vi "Y Translation Test.vi"() -> ()   [LabVIEW 2020]
doc: "This example performs writes and reads on a serial port, as directed by the user. You can press the Write and Read buttons, and change the Read Count, while the example is running.\n\nThe parameters set for the serial port must match the parameters of the connected instrument or device. In this example, the Read Count parameter specifies the number of bytes that the serial port reads. If there were more bytes at the port than the specified number, those bytes would not be read. If there were less bytes at the port than the specified number, you would receive a timeout error.\n\nThis example expands upon the flow control options for XON and XOFF, allowing the user to choose those control characters. Also, the user can enable or disable a termination character. Some devices require a termination character in order to identify the end of command strings. Some devices send a termination character to signify the end of data to be read. This example shows how you can end the Read operation once a termination character is detected in the buffer and/or append a termination character at the end of the Write data."
uses:
  Program Files/National Instruments/LabVIEW 2020/examples/Instrument IO/Serial/support/Serial - Settings.ctl
  <vilib>/Instr/_visa.llb/VISA Configure Serial Port (Instr).vi
panel:
  out "read buffer":string
  out "Limit Switch Activated":bool
  out "Moving":bool
  out "Boolean array":bool[](array[boolean])
  out "Number":i32
  out "Binary Number":i32=2374 format="%b"
  in  "Stop":bool
  in  "Command":string="@01 AMOV 200"
  in  "Send":bool
  in  "Serial Settings":T1={"baud rate"=57600, "data bits"=8, "parity"=enum."None", "stop bits"=10, "flow control"=0} {"flow control" items=["None"=0, "XON/XOFF"=1, "RTS/CTS"=2, "DTR/DSR"=4]; "stop bits" items=["1.0"=10, "1.5"=15, "2.0"=20]; "data bits" min=5 max=8 step=1; "baud rate" items=["75"=75, "110"=110, "134"=134, "150"=150, "300"=300, "600"=600, "1200"=1200, "1800"=1800, "2400"=2400, "4800"=4800, "7200"=7200, "9600"=9600, "14400"=14400, "19200"=19200, "28800"=28800, "38400"=38400, "56000"=56000, "57600"=57600, "115200"=115200, "128000"=128000, "230400"=230400]}
  in  "VISA resource name":refnum<visa-resource-name>="COM3"
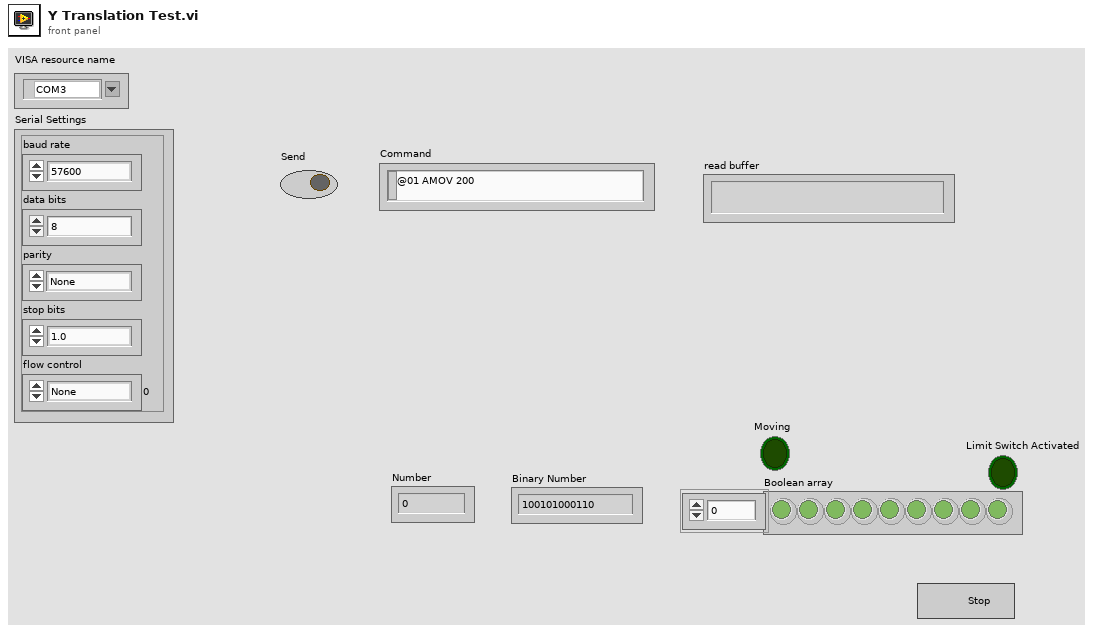
[diagram p1: front panel]
types:
  T1 = typedef "Serial - Settings.ctl" = cluster{"baud rate":u32, "data bits":u16, "parity":enum16{"None", "Odd", "Even", "Mark", "Space"}, "stop bits":u16, "flow control":u16}
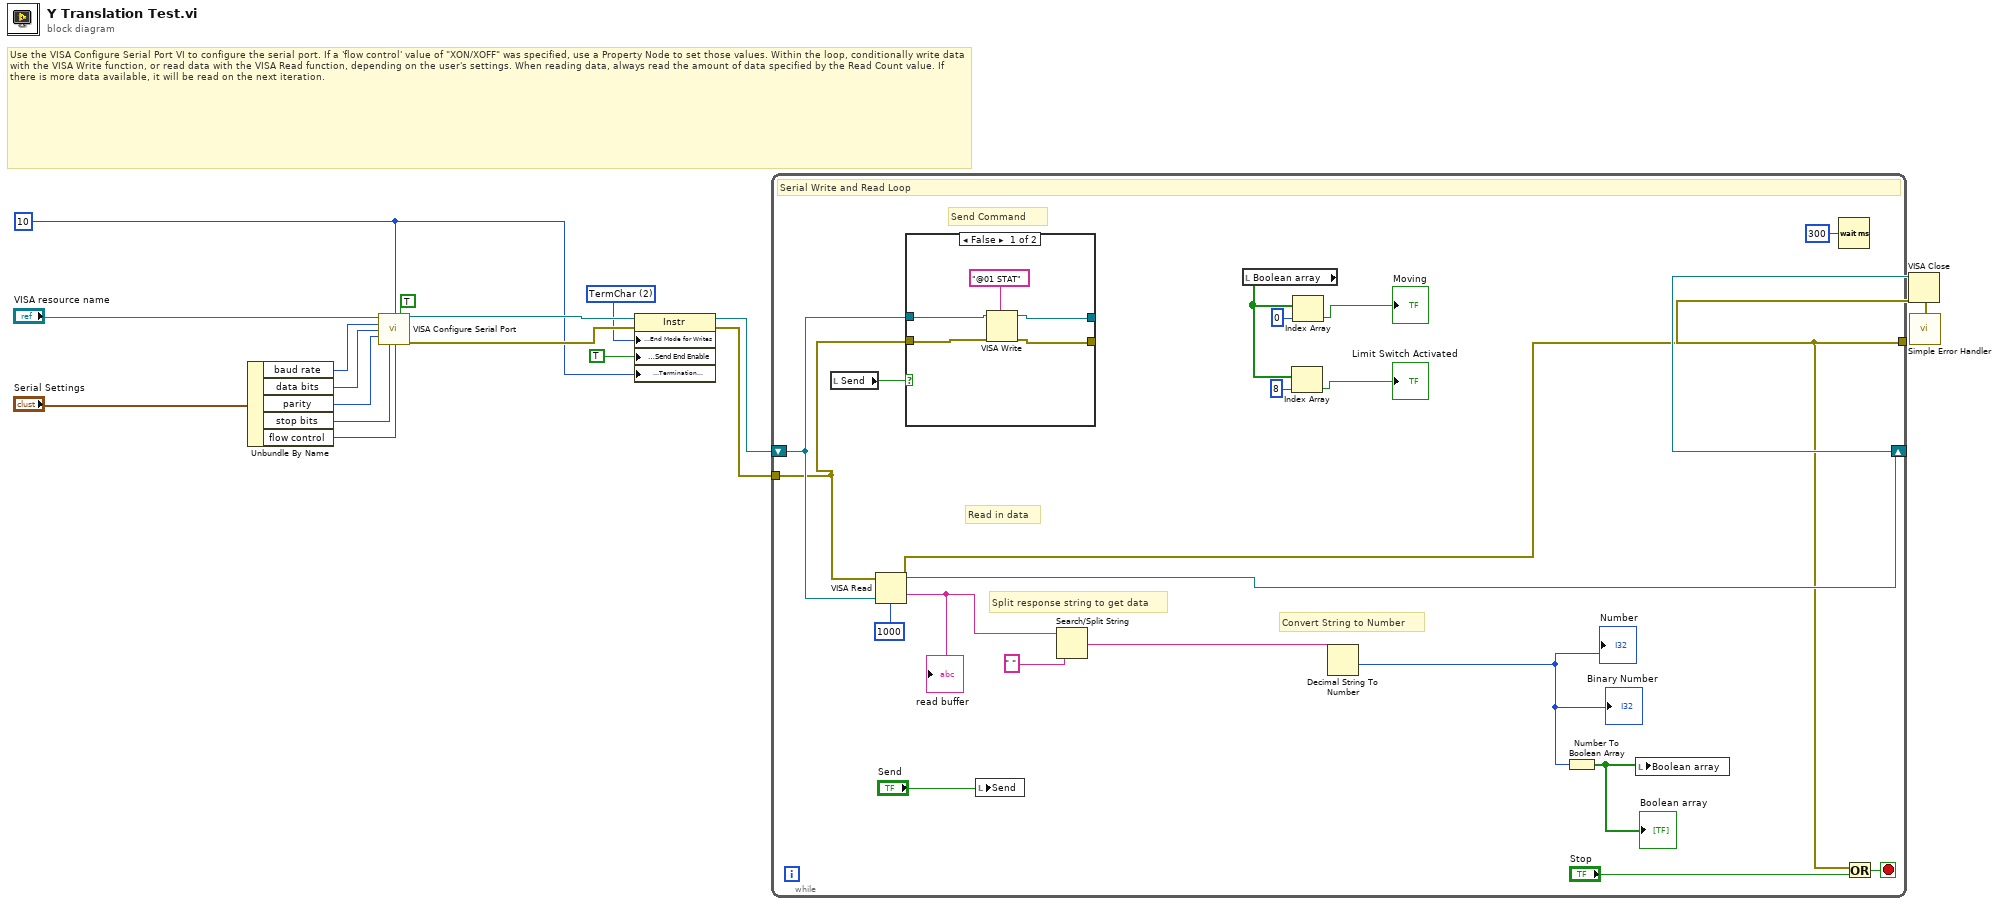
[diagram p0: block diagram]
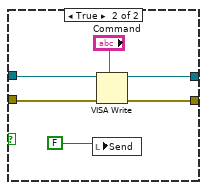
[diagram p2: hidden frame]
diagram:
  w1 = u8 10 ("Termination Character")
  w3 = u16 2 items=["None", "LastBit", "TermChar", "Break"] ("Serial Settings:Serial End Mode for Writes")
  # "Use the VISA Configure Serial Port VI to configure the serial port. If a 'flow control' value of \"XON/XOFF\" was specified, use a Property Node to set those values. Within the loop, conditionally write data with the VISA Write function, or read data with the VISA Read function, depending on the user's settings. When reading data, always read the amount of data specified by the Read Count value. If there is more data available, it will be read on the next iteration."
  n1 = Unbundle By Name("Serial Settings") -> ("baud rate"=w14:u32, "data bits"=w15:u16, "parity"=w16:enum16{"None", "Odd", "Even", "Mark", "Space"}, "stop bits"=w17:u16, "flow control"=w9:u16)
  n2 = call-poly "VISA Configure Serial Port"("VISA resource name"="VISA resource name", "termination char\n(0xA = '\\n' = LF)"=w1, "Enable Termination\nChar (T)"=TRUE ("End Read on Termination Character?"), "baud rate (9600)"=w14, "data bits (8)"=w15, "parity (0:none)"=w16, "stop bits (10: 1 bit)"=w17, "flow control (0:none)"=w9) -> ("VISA resource name out"=w6:refnum<visa-resource-name>, "error out"=w5:errorcluster)  [unwired: 2 in, 4 out]
  n3 = property class="Instr"(reference=w6, error in=w5, "Serial Settings:End Mode for Writes"=w3, "Message Based Settings:Send End Enable"=TRUE, "Message Based Settings:Termination Character"=w1) -> (reference out=w7:refnum<visa-resource-name>, error out=w8:errorcluster)
  n4 = while {
    shift-right: [w38] -> w10
    shift-left: w7 -> [w21]
    tunnel: w8 -> [w20]
    tunnel: [w35] -> w11
    stop <- w36 stop-if-true
    # "Send Command"
    # "Convert String to Number"
    # "Split response string to get data"
    # "Read in data"
    # "Serial Write and Read Loop"
    n5 = local read "Send"() -> (w22:bool)
    n6 = VISA Read(VISA resource name=w21, byte count=u32 1000 ("Read Word Length Count?"), error in (no error)=w20) -> (VISA resource name out=w38:refnum<visa-resource-name>, read buffer=w28:string, error out=w35:errorcluster)  [unwired: 1 out]
    "read buffer" <- w28
    n7 = case shown="False" w22 {
      tunnel: w21 -> [w43 w48]
      tunnel: w20 -> [w40 w47]
      tunnel: [w42 w46] -> _
      tunnel: [w41 w45] -> _
      frame False {
        n8 = VISA Write(VISA resource name=w43, write buffer="@01 STAT" ("Command 2"), error in (no error)=w40) -> (VISA resource name out=w42:refnum<visa-resource-name>, error out=w41:errorcluster)  [unwired: 1 out]
      }
      frame True {
        n9 = local write "Send"(FALSE) -> ()
        n10 = VISA Write(VISA resource name=w48, write buffer="Command", error in (no error)=w47) -> (VISA resource name out=w46:refnum<visa-resource-name>, error out=w45:errorcluster)  [unwired: 1 out]
      }
    }
    n11 = local write "Send"("Send") -> ()
    n12 = Search/Split String(string=w28, search string/char (-)=" ") -> (match + rest of string=w26:string)  [unwired: 1 in, 2 out]
    n13 = local read "Boolean array"() -> (w31:bool[])
    n14 = Index Array(array=w31, index=8) -> (element=→"Limit Switch Activated":bool)
    n15 = Index Array(array=w31, index=0) -> (element=→"Moving":bool)
    n16 = Decimal String To Number(string=w26) -> (number=w24:i32)  [unwired: 2 in, 1 out]
    "Binary Number" <- w24
    "Number" <- w24
    n17 = Number To Boolean Array(number=w24) -> (Boolean array=w23:bool[])
    "Boolean array" <- w23
    n18 = local write "Boolean array"(w23) -> ()
    n19 = Wait (ms)(milliseconds to wait=u32 300) -> ()  [unwired: 1 out]
    n20 = Or(x=w35, y="Stop") -> (x .or. y?=w36:bool)
  }
  n21 = VISA Close(VISA resource name=w10, error in (no error)=w11) -> (error out=w12:errorcluster)
  n22 = call <vilib>:"Simple Error Handler.vi"("error in (no error)"=w12) -> ()  [unwired: 1 in, 8 out]
